vi "test-traj-generate-0-way.vi"() -> ()   [LabVIEW 2019]
uses:
  <vilib>/Rock Robotics/WPI/ThirdParty/JAS_Junk/TrajLib/Trajectory_Library.lvlib
  <vilib>/Rock Robotics/WPI/ThirdParty/JAS_Junk/TrajLib/TypeDef/TRANSLATION2D.ctl
  <vilib>/Rock Robotics/WPI/ThirdParty/JAS_Junk/TrajLib/TypeDef/ROTATION2D.ctl
  <vilib>/Rock Robotics/WPI/ThirdParty/JAS_Junk/TrajLib/TypeDef/POSE2D.ctl
  <vilib>/Rock Robotics/WPI/ThirdParty/JAS_Junk/TrajLib/TypeDef/TRAJ_CONFIG.ctl
  <vilib>/Analysis/Matrix/Datatypes/RealMatrix.ctl
  <vilib>/Analysis/Matrix/NI_Matrix.lvlib
  <vilib>/Rock Robotics/WPI/ThirdParty/JAS_Junk/TrajLib/TypeDef/POSEwCURVATURE.ctl
  <vilib>/Rock Robotics/WPI/ThirdParty/JAS_Junk/TrajLib/TypeDef/SPLINE_CTRL_VECTOR.ctl
  <vilib>/Rock Robotics/WPI/ThirdParty/JAS_Junk/TrajLib/TypeDef/TRAJECTORY.ctl
  <vilib>/Rock Robotics/WPI/ThirdParty/JAS_Junk/TrajLib/TypeDef/TRAJ_STATE.ctl
  <vilib>/Rock Robotics/WPI/ThirdParty/JAS_Junk/TrajLib/TypeDef/SPLINE.ctl
  <vilib>/Rock Robotics/WPI/ThirdParty/JAS_Junk/TrajLib/TypeDef/DISPLAY_WAYPOINT.ctl
panel:
  in  "Tab Control":T1(tab)
  in  "InteriorWayPoints":T2[](array[typedef]) {"Y" format="%14.3f"; "X" format="%14.3f"}
  in  "Initial_Position":T3={"X"=0.0, "Y"=-2.0, "ANGLE"=0.0} {"ANGLE" format="%13.3f"; "Y" format="%13.3f"; "X" format="%13.3f"}
  in  "Ending_Position":T3={"X"=2.0, "Y"=0.0, "ANGLE"=1.57} {"ANGLE" format="%13.3f"; "Y" format="%13.3f"; "X" format="%13.3f"}
  out "initialSpline_Ctrl_Vector":T4
  out "endSpline_Ctrl_Vector":T4
  out "splines":T5[](array[typedef])
  out "ArrayPoseWithCurvature":T7[](array[typedef]) {"POSE"."ROTATION"."SIN" format="%13.4f"; "POSE"."ROTATION"."COS" format="%13.4f"; "POSE"."ROTATION"."VALUE" format="%13.4f"; "POSE"."TRANSLATION"."Y" format="%14.3f"; "POSE"."TRANSLATION"."X" format="%14.3f"}
  out "PoseCSize":i32
  out "error out 2":errorcluster
  in  "Config":T10={"MaxVelocity"=2.0, "Max Acceleration"=2.0, "StartVelocity"=0.0, "End Velocity"=0.0, "Reversed"=FALSE, "Constraints"=[]} {"End Velocity" format="%20.4f"; "StartVelocity" format="%20.4f"; "Max Acceleration" format="%20.4f"; "MaxVelocity" format="%20.4f"}
  out "TRAJECTORY":T11 {"States"."POSE"."ROTATION"."SIN" format="%13.4f"; "States"."POSE"."ROTATION"."COS" format="%13.4f"; "States"."POSE"."ROTATION"."VALUE" format="%13.4f"; "States"."POSE"."TRANSLATION"."Y" format="%14.3f"; "States"."POSE"."TRANSLATION"."X" format="%14.3f"; "TotalTImeSecs" format="%20.3f"}
  out "size(s)":i32
  out "error out":errorcluster
  out "XY Graph":cluster{dbl[], dbl[]}(graph)
  out "Position":cluster{dbl[], dbl[]}(graph)
  out "Done":bool
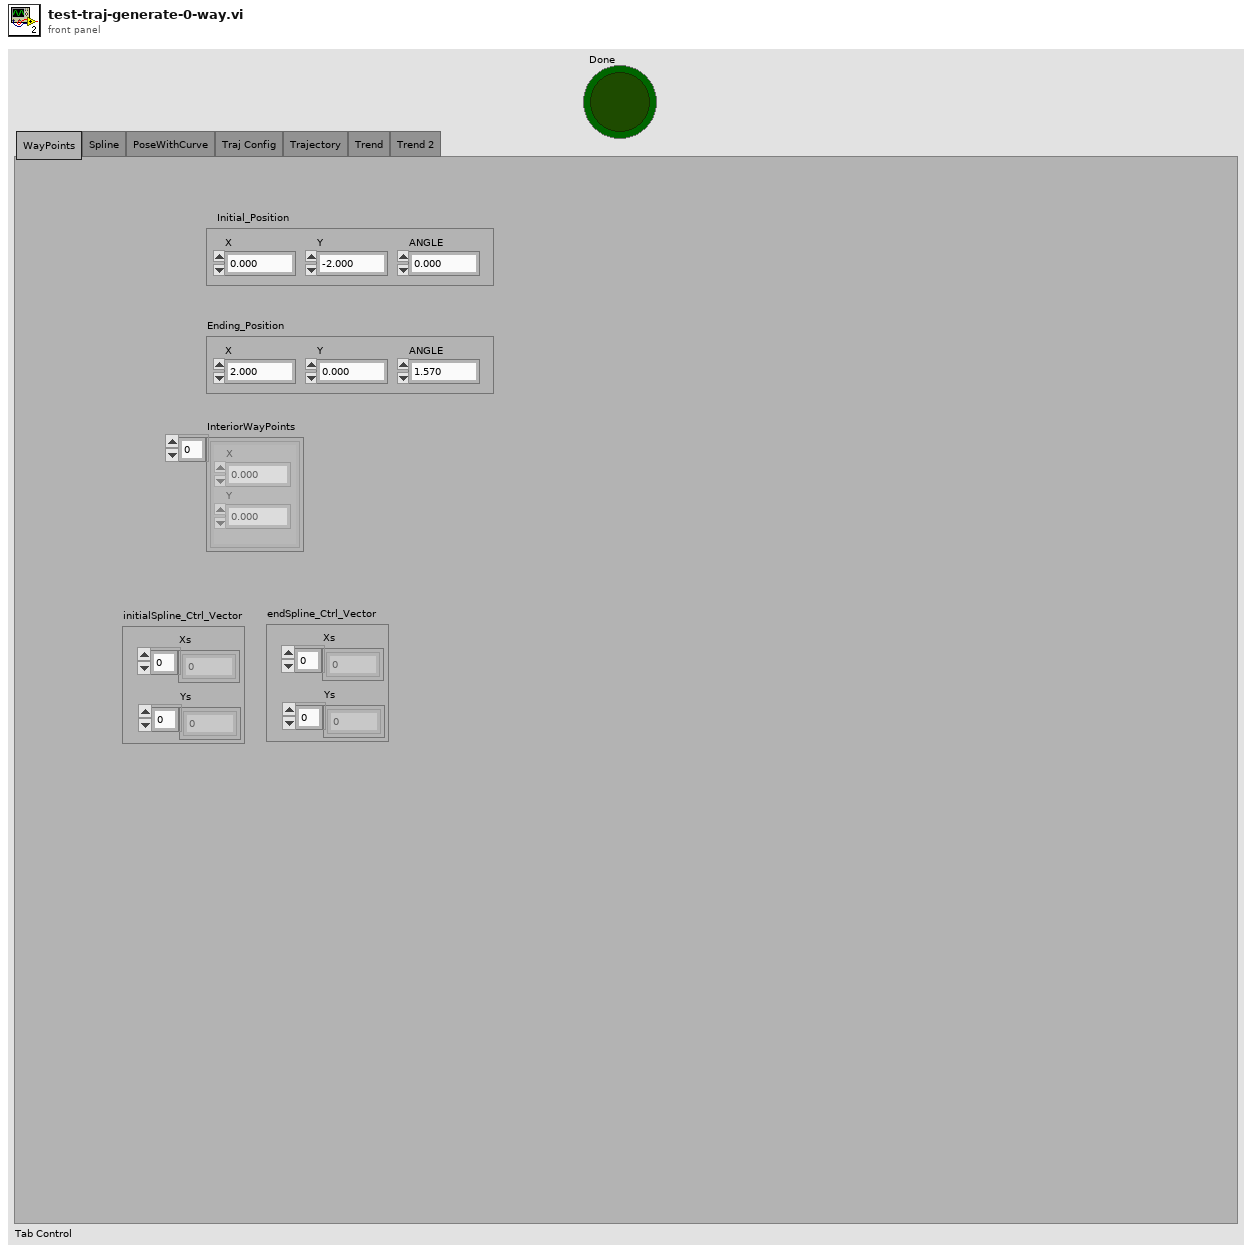
[diagram p1: front panel]
types:
  T1 = enum32{"WayPoints", "Spline", "PoseWithCurve", "Traj Config", "Trajectory", "Trend", "Trend 2"}
  T2 = typedef "Trajectory_Library.lvlib/TRANSLATION2D.ctl" = cluster{"X":dbl, "Y":dbl}
  T3 = typedef "Trajectory_Library.lvlib/DISPLAY_WAYPOINT.ctl" = cluster{"X":dbl, "Y":dbl, "ANGLE":dbl}
  T4 = typedef "Trajectory_Library.lvlib/SPLINE_CTRL_VECTOR.ctl" = cluster{"Xs":dbl[], "Ys":dbl[]}
  T5 = typedef "Trajectory_Library.lvlib/SPLINE.ctl" = cluster{"Degree":i32, "Coefficients":T6}
  T6 = typedef "NI_Matrix.lvlib/RealMatrix.ctl" = dbl[][]
  T7 = typedef "Trajectory_Library.lvlib/POSEwCURVATURE.ctl" = cluster{"CURVATURE":dbl, "POSE":T8}
  T8 = typedef "Trajectory_Library.lvlib/POSE2D.ctl" = cluster{"TRANSLATION":T2, "ROTATION":T9}
  T9 = typedef "Trajectory_Library.lvlib/ROTATION2D.ctl" = cluster{"VALUE":dbl, "COS":dbl, "SIN":dbl}
  T10 = typedef "Trajectory_Library.lvlib/TRAJ_CONFIG.ctl" = cluster{"MaxVelocity":dbl, "Max Acceleration":dbl, "StartVelocity":dbl, "End Velocity":dbl, "Reversed":bool, "Constraints":variant[]}
  T11 = typedef "Trajectory_Library.lvlib/TRAJECTORY.ctl" = cluster{"TotalTImeSecs":dbl, "States":T12[]}
  T12 = typedef "Trajectory_Library.lvlib/TRAJ_STATE.ctl" = cluster{"TimeSeconds":dbl, "Velocity":dbl, "Acceleration":dbl, "POSE":T8, "Curvature":dbl}
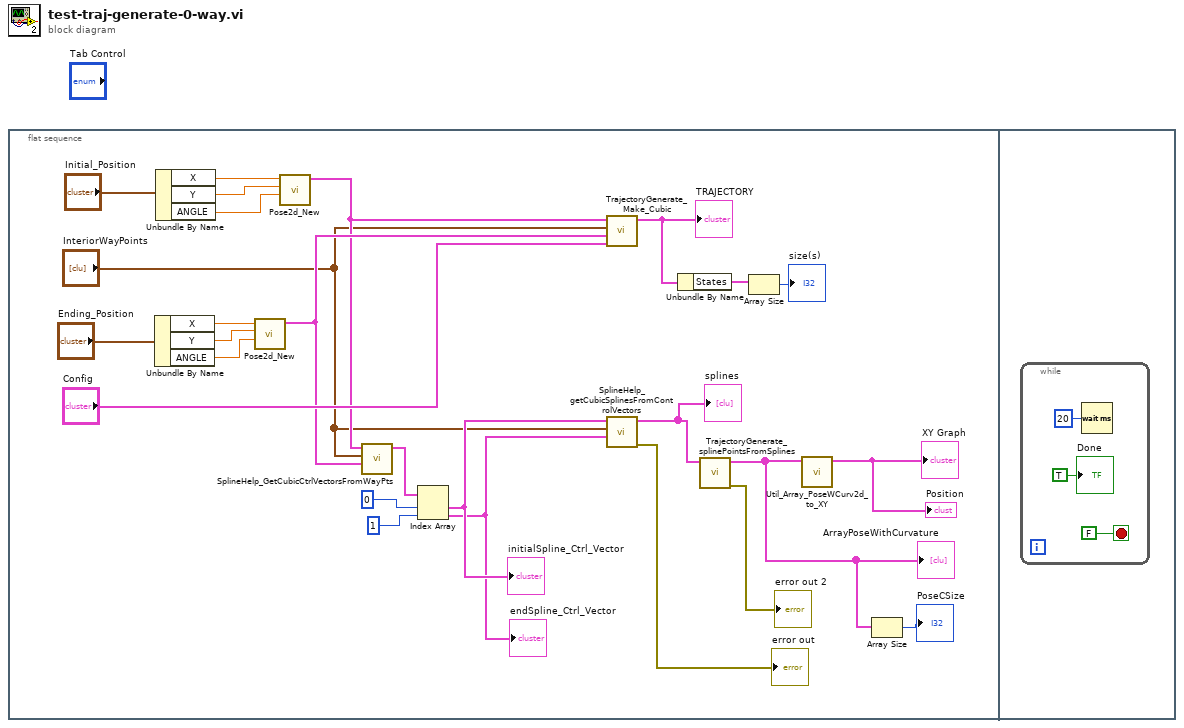
[diagram p0: block diagram]
diagram:
  n1 = flat-sequence {
    frame #0 {
      n2 = Unbundle By Name("Ending_Position") -> ("X"=w21:dbl, "Y"=w20:dbl, "ANGLE"=w19:dbl)
      n3 = Unbundle By Name("Initial_Position") -> ("X"=w24:dbl, "Y"=w23:dbl, "ANGLE"=w22:dbl)
      n4 = call <vilib>:"Pose2d_New.vi"("Heading"=w19, "Y"=w20, "X"=w21) -> ("out POSe"=w17:T8)  [unwired: 8 in]
      n5 = call <vilib>:"Pose2d_New.vi"("Heading"=w22, "Y"=w23, "X"=w24) -> ("out POSe"=w16:T8)  [unwired: 8 in]
      n6 = call <vilib>:"SplineHelp_GetCubicCtrlVectorsFromWayPts.vi"("Enging POSE"=w17, "Interior WAYPOINTS"="InteriorWayPoints", "Starting POSE"=w16) -> ("SplineControlVectors"=w5:T4[])  [unwired: 8 in]
      n7 = Index Array(array=w5, index #1=0 ("index"), index #2=1 ("index")) -> (element #1=w4:T4, element #2=w3:T4)
      "initialSpline_Ctrl_Vector" <- w4
      "endSpline_Ctrl_Vector" <- w3
      n8 = call <vilib>:"TrajectoryGenerate_Make_Cubic.vi"("traj_config"="Config", "Enging POSE"=w17, "Interior WAYPOINTS"="InteriorWayPoints", "Starting POSE"=w16) -> ("TRAJECTORY"=w12:T11)  [unwired: 6 in, 1 out]
      "TRAJECTORY" <- w12
      n9 = call <vilib>:"SplineHelp_getCubicSplinesFromControlVectors.vi"("endCtrlVector"=w3, "InternalWaypoints"="InteriorWayPoints", "startCtrlVector"=w4) -> ("error out"=→"error out":errorcluster, "splines"=w14:T5[])  [unwired: 3 in, 4 out]
      "splines" <- w14
      n10 = Unbundle By Name(w12) -> ("States"=w11:T12[])
      n11 = call <vilib>:"TrajectoryGenerate_splinePointsFromSplines.vi"("inputSPLINE"=w14) -> ("error out"=→"error out 2":errorcluster, "ArrayPoseWithCurvature"=w2:T7[])  [unwired: 9 in]
      "ArrayPoseWithCurvature" <- w2
      n12 = Array Size(array=w11) -> (size(s)=→"size(s)":i32)
      n13 = call <vilib>:"Util_Array_PoseWCurv2d_to_XY.vi"("inArrayPoseWCurve"=w2) -> ("outArrayXY"=→"XY Graph" →"Position":cluster{dbl[], dbl[]})  [unwired: 10 in]
      n14 = Array Size(array=w2) -> (size(s)=→"PoseCSize":i32)
    }
    frame #1 {
      n15 = while {
        stop <- FALSE stop-if-true
        n16 = Wait (ms)(milliseconds to wait=u32 20) -> ()  [unwired: 1 out]
        "Done" <- TRUE ("Done")
      }
    }
  }
